vi "Command Stop Model.vi"(8 "Password":string, 9 "Username":string, 11 "Target IP Address":string="10.0.35.19") -> (0 "error out":errorcluster)   [LabVIEW 2020]
uses:
  Web Service/Endpoints.ctl
  <vilib>/httpClient/LabVIEWHTTPClient.lvlib
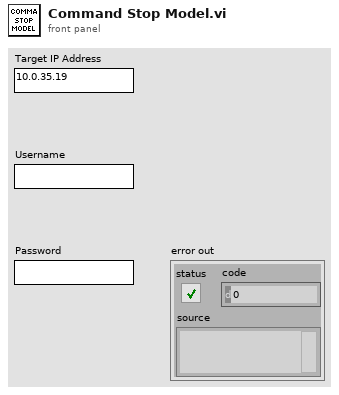
[diagram p1: front panel]
types:
  T1 = typedef "Endpoints.ctl" = string
  T2 = typedef "LabVIEWHTTPClient.lvlib/ClientHandle.ctl" = refnum<k1>
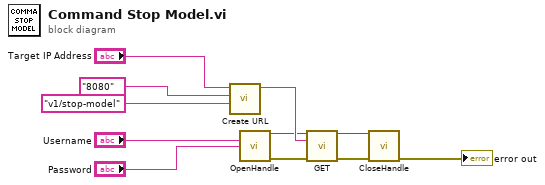
[diagram p0: block diagram]
diagram:
  n1 = call "Create URL.vi"("endpoint"=T1 "v1/stop-model", "port"="8080", "Target IP Address"="Target IP Address") -> ("URL Out"=w10:string)  [unwired: 8 in]
  n2 = call <vilib>:"OpenHandle.vi"("username"="Username", "password"="Password") -> ("client handle out"=w2:T2, "error out"=w1:errorcluster)  [unwired: 12 in]
  n3 = call <vilib>:"GET.vi"("client handle"=w2, "url"=w10, "error in (no error)"=w1) -> ("client handle out"=w4:T2, "error out"=w3:errorcluster)  [unwired: 9 in, 2 out]
  n4 = call <vilib>:"CloseHandle.vi"("client handle"=w4, "error in (no error)"=w3) -> ("error out"=→"error out":errorcluster)  [unwired: 13 in]
